vi "EnqueError.vi"(7 "QueName":string="BaseVisQue", 8 "Error":errorcluster[](array[cluster])) -> (0 "Error":errorcluster[](array[cluster]))   [LabVIEW 2014, in "Visualization.lvlib" / "VisualizeBase.lvclass"]
uses:
  VisualizeBase/VisualizeBase_class/VisualizeBase.lvclass
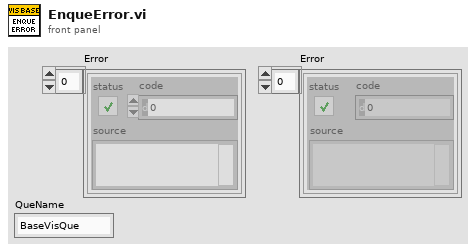
[diagram p1: front panel]
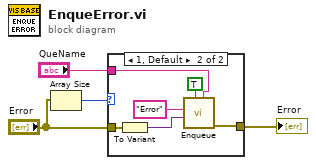
[diagram p0: block diagram]
diagram:
  n1 = Array Size(array="Error") -> (size(s)=w4:i32)
  n2 = case shown="1, Default" w4 {
    tunnel: [w5 w9] -> w2
    tunnel: "Error" -> [w5 w11]
    tunnel: "QueName" -> [_ w6]
    frame 0 {
    }
    frame 1, Default {
      n3 = To Variant(anything=w11) -> (Variant=w10:variant)
      n4 = call "Enqueue.vi"("QueName"=w6, "Priority? (F)"=TRUE, "Data"=w10, "Message"="Error") -> ("Error"=w9:errorcluster[])  [unwired: 7 in]
    }
  }
  "Error" <- w2
